vi "Get Value (String).vi"(8 "error in":errorcluster, 10 "TPCANParameter":T2, 11 "TPCANHandle in":T1 items=["PCAN_NONEBUS"=0, "PCAN_USBBUS1"=81, "PCAN_USBBUS2"=82, "PCAN_USBBUS3"=83, "PCAN_USBBUS4"=84, "PCAN_USBBUS5"=85, "PCAN_USBBUS6"=86, "PCAN_USBBUS7"=87, "PCAN_USBBUS8"=88, "PCAN_USBBUS9"=1289, "PCAN_USBBUS10"=1290, "PCAN_USBBUS11"=1291, "PCAN_USBBUS12"=1292, "PCAN_USBBUS13"=1293, "PCAN_USBBUS14"=1294, "PCAN_USBBUS15"=1295, "PCAN_USBBUS16"=1296]) -> (0 "error out":errorcluster, 1 "Value":string, 3 "TPCANHandle out":T1 items=["PCAN_NONEBUS"=0, "PCAN_USBBUS1"=81, "PCAN_USBBUS2"=82, "PCAN_USBBUS3"=83, "PCAN_USBBUS4"=84, "PCAN_USBBUS5"=85, "PCAN_USBBUS6"=86, "PCAN_USBBUS7"=87, "PCAN_USBBUS8"=88, "PCAN_USBBUS9"=1289, "PCAN_USBBUS10"=1290, "PCAN_USBBUS11"=1291, "PCAN_USBBUS12"=1292, "PCAN_USBBUS13"=1293, "PCAN_USBBUS14"=1294, "PCAN_USBBUS15"=1295, "PCAN_USBBUS16"=1296], 5 "TPCANStatus":u32)   [LabVIEW 2020, in "PCANBasic.lvlib"]
uses:
  PCANBasic.lvlib
  peak/PCANBasic64.dll
  TPCANParameter.ctl
  TPCANHandle.ctl
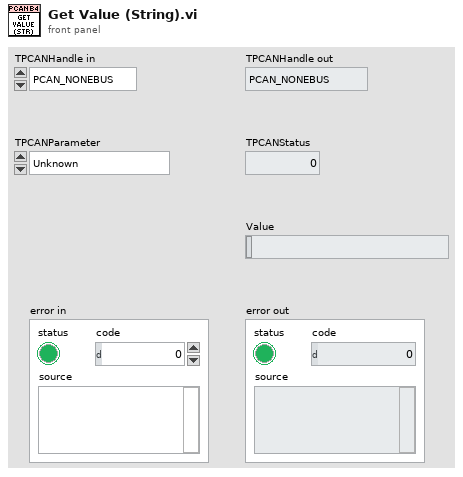
[diagram p1: front panel]
types:
  T1 = typedef "PCANBasic.lvlib/TPCANHandle.ctl" = u16
  T2 = typedef "PCANBasic.lvlib/TPCANParameter.ctl" = enum8{"Unknown", "PCAN_DEVICE_ID", "PCAN_5VOLTS_POWER", "PCAN_RECEIVE_EVENT", "PCAN_MESSAGE_FILTER", "PCAN_API_VERSION", "PCAN_CHANNEL_VERSION", "PCAN_BUSOFF_AUTORESET", "PCAN_LISTEN_ONLY", "PCAN_LOG_LOCATION", "PCAN_LOG_STATUS", "PCAN_LOG_CONFIGURE", "PCAN_LOG_TEXT", "PCAN_CHANNEL_CONDITION", "PCAN_HARDWARE_NAME", "PCAN_RECEIVE_STATUS", "PCAN_CONTROLLER_NUMBER", "PCAN_TRACE_LOCATION", "PCAN_TRACE_STATUS", "PCAN_TRACE_SIZE", "PCAN_TRACE_CONFIGURE", "PCAN_CHANNEL_IDENTIFYING", "PCAN_CHANNEL_FEATURES", "PCAN_BITRATE_ADAPTING", "PCAN_BITRATE_INFO", "PCAN_BITRATE_INFO_FD", "PCAN_BUSSPEED_NOMINAL", "PCAN_BUSSPEED_DATA", "PCAN_IP_ADDRESS", "PCAN_LAN_SERVICE_STATUS", "PCAN_ALLOW_STATUS_FRAMES", "PCAN_ALLOW_RTR_FRAMES", "PCAN_ALLOW_ERROR_FRAMES", "PCAN_INTERFRAME_DELAY", "PCAN_ACCEPTANCE_FILTER_11BIT", "PCAN_ACCEPTANCE_FILTER_29BIT", "PCAN_IO_DIGITAL_CONFIGURATION", "PCAN_IO_DIGITAL_VALUE", "PCAN_IO_DIGITAL_SET", "PCAN_IO_DIGITAL_CLEAR", "PCAN_IO_ANALOG_VALUE", "PCAN_FIRMWARE_VERSION", "PCAN_ATTACHED_CHANNELS_COUNT", "PCAN_ATTACHED_CHANNELS", "PCAN_ALLOW_ECHO_FRAMES", "PCAN_DEVICE_PART_NUMBER", "PCAN_HARD_RESET_STATUS", "PCAN_LAN_CHANNEL_DIRECTION", "PCAN_DEVICE_GUID"}
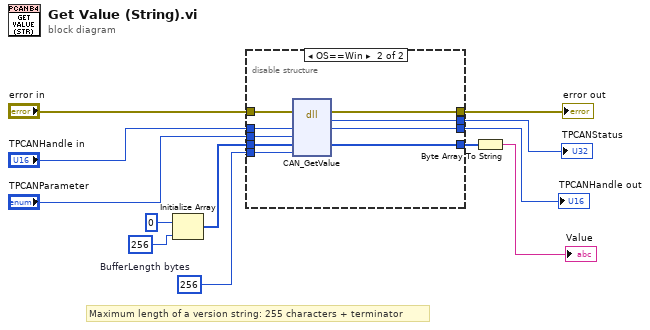
[diagram p0: block diagram]
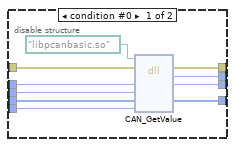
[diagram p2: hidden frame]
diagram:
  w6 = u32 256  # BufferLength bytes
  # "Maximum length of a version string: 255 characters + terminator"
  n1 = Initialize Array(u8 0 ("char"), 256 ("dimension size")) -> (w10:u8[])
  n2 = disable-structure shown="OS==Win" {
    disable-tunnel: "TPCANHandle in" -> [w22 w31]
    disable-tunnel: "error in" -> [w21 w30]
    disable-tunnel: [w20 w29] -> w4
    disable-tunnel: "TPCANParameter" -> [w19 w28]
    disable-tunnel: w6 -> [w18 w27]
    disable-tunnel: [w17 w26] -> w7
    disable-tunnel: w10 -> [w16 w25]
    disable-tunnel: [w15 w24] -> w12
    disable-tunnel: [w13 w23] -> w1
    frame condition #0 {
      n3 = dll-call lib="?" fn="CAN_GetValue"(path in=path "libpcanbasic.so", error in=w21, "Channel"=w22, "TPCANParameter"=w19, "Buffer"=w16, "BufferLength"=w18) -> (error out=w20:errorcluster, "TPCANStatus"=w17:u32, "Channel"=w13:u16, "Buffer"=w15:u8[])  [unwired: 3 in, 1 out]
    }
    frame condition #1 (active) {
      n4 = dll-call lib="D:/git/PCAN-Basic-LabVIEW/source/peak/PCANBasic*.dll" fn="CAN_GetValue"(error in=w30, "Channel"=w31, "TPCANParameter"=w28, "Buffer"=w25, "BufferLength"=w27) -> (error out=w29:errorcluster, "TPCANStatus"=w26:u32, "Channel"=w23:u16, "Buffer"=w24:u8[])  [unwired: 4 in, 1 out]
    }
  }
  "TPCANStatus" <- w7
  "error out" <- w4
  "TPCANHandle out" <- w1
  n5 = Byte Array To String(unsigned byte array=w12) -> (string=→"Value":string)
